vi "Append VI Hierarchy to Report (string).vi"(0 "report in":refnum<class "NI_report.lvclass">, 2 "image format (jpeg)":enum32{"PNG", "JPEG", "GIF"}(ring)=enum."JPEG", 5 "VI":string, 7 "alignment (default)":T2, 11 "error in (no error)":errorcluster, 12 "MS Office parameters":T1) -> (4 "report out":refnum<class "NI_report.lvclass">, 6 "VI name out":string, 8 "start out (Word)":i32, 10 "end out (Word)":i32, 15 "error out":errorcluster)   [LabVIEW 2020, in "NI_ReportGenerationCore.lvlib"]
doc: "Appends the hierarchy of the VI you specify in <B>VI</B> to a report. Wire data to the <B>VI</B> input to determine the polymorphic instance to use or manually select the instance."
uses:
  <vilib>/Utility/NIReport.llb/NI_ReportGenerationCore.lvlib
  <vilib>/Utility/NIReport.llb/NI_report.lvclass
  <vilib>/Utility/NIReport.llb/HTML Report Image Alignment.ctl
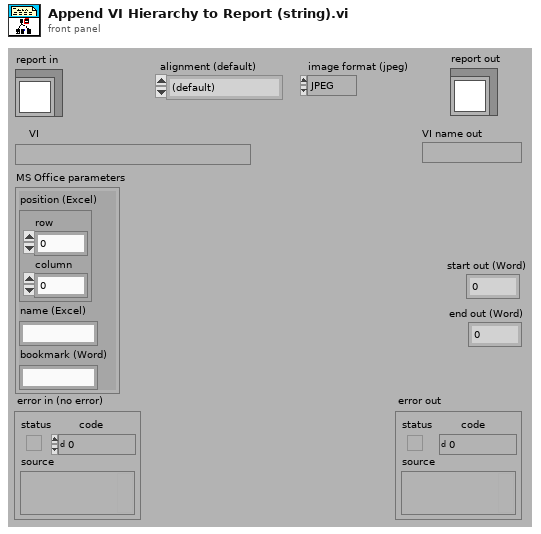
[diagram p1: front panel]
types:
  T1 = cluster{"position (Excel)":cluster{"row":i32, "column":i32}, "name (Excel)":string, "bookmark (Word)":string}
  T2 = typedef "NI_ReportGenerationCore.lvlib/HTML Report Image Alignment.ctl" = enum16{"(default)", "LEFT", "RIGHT", "TOP", "TEXTTOP", "MIDDLE", "ABSMIDDLE", "BASELINE", "BOTTOM", "ABSBOTTOM"}
  T3 = enum32{"invalid app kind", "Development System", "Run Time System", "Student Edition", "Embedded LabVIEW", "Evaluation", "Custom"}
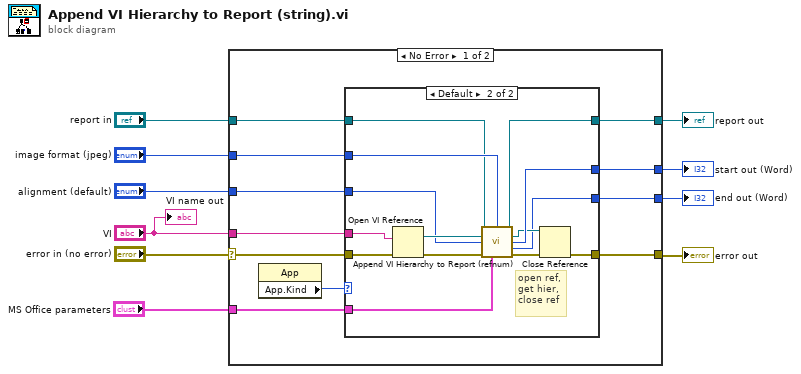
[diagram p0: block diagram]
diagram:
  n1 = case shown="No Error" "error in (no error)" {
    selector: "error in (no error)" -> [w20 w39]
    tunnel: [w16 w39] -> w9
    tunnel: [w14 w38] -> w7
    tunnel: "report in" -> [w13 w38]
    tunnel: "VI" -> [w21 _]
    tunnel: "image format (jpeg)" -> [w17 _]
    tunnel: "MS Office parameters" -> [w19 _]
    tunnel: "alignment (default)" -> [w18 _]
    tunnel: [w15 _] -> w2
    tunnel: [w12 _] -> w1
    frame No Error {
      n2 = property class="App"() -> ("App.Kind"=w11:T3)  [unwired: 2 in, 2 out]
      n3 = case shown="Default" w11 {
        tunnel: w21 -> [_ w37]
        tunnel: w20 -> [w23 w36]
        tunnel: w19 -> [_ w33]
        tunnel: w18 -> [_ w32]
        tunnel: w17 -> [_ w31]
        tunnel: [w23 w29] -> w16
        tunnel: [_ w28] -> w15
        tunnel: [w22 w27] -> w14
        tunnel: w13 -> [w22 w26]
        tunnel: [_ w24] -> w12
        frame "Run Time System" {
          # "Do not try to append\nif running in an\nexecutable"
        }
        frame Default {
          # "open ref,\nget hier,\nclose ref"
          n4 = Open VI Reference(vi path=w37, error in (no error)=w36) -> (vi reference=w35:refnum<vi>, error out=w34:errorcluster)  [unwired: 4 in]
          n5 = call <vilib>:"Append VI Hierarchy to Report (refnum).vi"("report in"=w26, "image format (jpeg)"=w31, "VI"=w35, "alignment (default)"=w32, "error in (no error)"=w34, "MS Office parameters"=w33) -> ("report out"=w27:refnum<class "NI_report.lvclass">, "VI out"=w25:refnum<vi>, "start out (Word)"=w28:i32, "end out (Word)"=w24:i32, "error out"=w30:errorcluster)  [unwired: 5 in]
          n6 = Close Reference(reference=w25, error in (no error)=w30) -> (error out=w29:errorcluster)
        }
      }
    }
    frame Error {
    }
  }
  "error out" <- w9
  "report out" <- w7
  "start out (Word)" <- w2
  "end out (Word)" <- w1
  "VI name out" <- "VI"
